vi "Check Alias Already Exists.vi"(9 "Alias":string, 10 "Actor":refnum<class "Actor.lvclass">) -> (2 "Error":errorcluster)   [LabVIEW 2020, in "jettl.lvlib"]
uses:
  jettl.lvlib
  Actor/Actor.lvclass
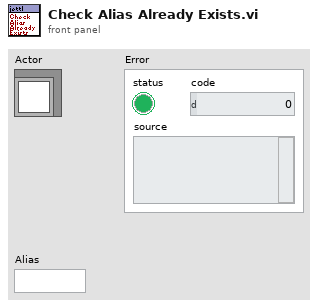
[diagram p1: front panel]
types:
  T1 = typedef "jettl.lvlib/Child Actor Attributes.ctl" = map{string, T2}
  T2 = typedef "jettl.lvlib/Actor Attributes.ctl" = cluster{"Unified Layer":T3, "Root":bool, "Alias":string, "UID":i32, "Transport":refnum<user-event>, "Address":refnum<event-registration>, "This VI":refnum<vi>}
  T3 = typedef "jettl.lvlib/Unified Layer.ctl" = cluster{"Msgs":T4, "Leaf":bool}
  T4 = typedef "jettl.lvlib/Msgs.ctl" = set{refnum<class "Msg.lvclass">}
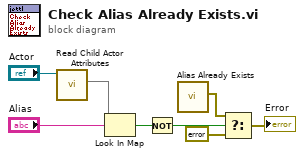
[diagram p0: block diagram]
diagram:
  n1 = call-dynamic "Read Child Actor Attributes.vi"("Actor in"="Actor") -> ("Child Actor Attributes"=w4:T1)  [unwired: 10 in]
  n2 = Look In Map(map=w4, key="Alias") -> (key not found?=w2:bool)  [unwired: 1 in, 1 out]
  n3 = Not(x=w2) -> (.not. x?=w1:bool)
  n4 = call "Alias Already Exists.vi"() -> ("Error"=w8:errorcluster)  [unwired: 11 in]
  n5 = Select(t=w8, s=w1, f=errorcluster {"status"=FALSE, "code"=0, "source"=""}) -> (s? t:f=→"Error":errorcluster)
